vi "Read_write_p4.vi"() -> ()   [LabVIEW 2018]
uses:
  <instrlib>/LeCroy Wave Series/Public/Data/Read Single Waveform.vi
  <vilib>/Utility/file.llb/Read Delimited Spreadsheet (DBL).vi
  <vilib>/Utility/file.llb/Write Delimited Spreadsheet (DBL).vi
  <instrlib>/Siglent SDG X Series/Siglent SDG X Series.lvlib
  <instrlib>/LeCroy Wave Series/LeCroy Wave Series.lvlib
panel:
  in  "#Iteration":i32
  out "path":path
  out "error out 5":errorcluster
  out "error out 4":errorcluster
  out "resulting string":string
  out "#N_packet":i32
  out "error IO 2":errorcluster
  out "error IO":errorcluster
  in  "Read Directory":string
  out "error out 3":errorcluster
  in  "Write Directory":string
  in  "N_packets":i32
  in  "all rows 1":dbl[](array[numeric])
  in  "Tab Control":enum32{"Page 1", "Page 2"}(tab)
  in  "VISA Refnum in":refnum<visa-resource-name>
  in  "error in (no error)":errorcluster
  in  "Channel (1:Channel 1)":i32(ring)=1 items=["Channel 1"=1, "Channel 2"=2]
  in  "Enable Output (T: Enable)":bool=TRUE
  in  "Amplitude (1.0 Vpp)":dbl=1.0 format="%#.3f"
  in  "Frequency (1000 Hz)":dbl=1000.0 format="%#.6g"
  in  "DC Offset (0.00 V) in":dbl
  in  "Waveform Function (0: Sine) in":u16(ring) items=["Sine", "Square", "Ramp", "DC", "Pulse", "Arb"]
  in  "Phase (0.0 degrees)":dbl=0.002 min=-360.0 max=360.0 format="%#.1g"
  in  "Fall (20 ns)":dbl=2e-08 format="%#.3g"
  in  "Duty (20%)":dbl=4.32 min=0.0001 max=100.0 format="%.4g"
  in  "Delay (0.00 s)":dbl min=-1000000.0 max=1000000.0
  in  "Rise (20 ns)":dbl=1.04e-08 format="%#.3g"
  in  "True To \ngenerate\n pulse":bool
  out "VISA resource name out":refnum<visa-resource-name>
  out "error out":errorcluster
  in  "format string":string
  out "Output Filename":path
  out "error out 2":errorcluster
  in  "Filename":string="filename"
  in  "Path":string="c:\\path structure\\"
  in  "Read Directory":string
  out "Waveform Data":waveform(dbl)(graph)
  in  "Timeout (10000 ms)":u32=10000
  in  "Source (0: Channel 1)":u16(ring) items=["Channel 1", "Channel 2", "Channel 3", "Channel 4", "Memory 1", "Memory 2", "Memory 3", "Memory 4", "Function 1", "Function 2", "Function 3", "Function 4", "Function 5", "Function 6", "Function 7", "Function 8"]
  in  "Perform Auto Setup?":bool
  in  "Reset Scope?":bool
  in  "VISA resource name":refnum<visa-resource-name>
  out "Saved filename":string
  # "Set PULSE parameters"
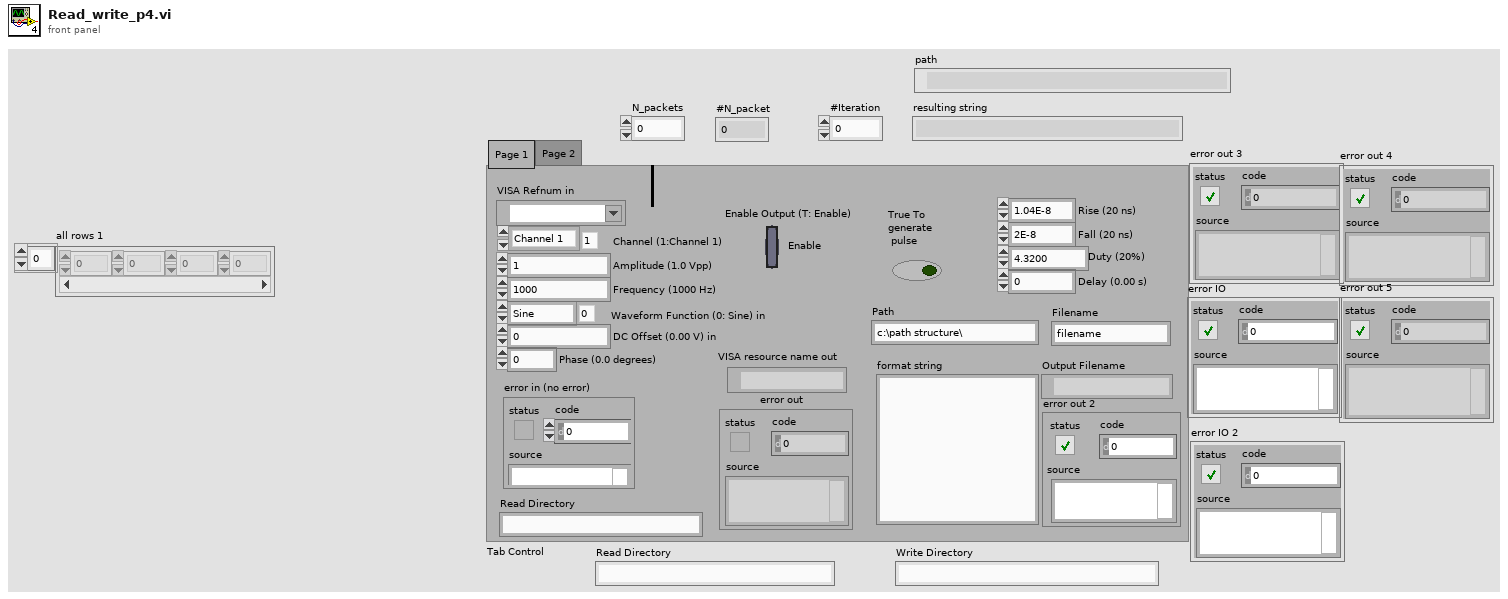
[diagram p1: front panel]
types:
  T1 = enum16{"open", "replace", "create", "open or create", "replace or create", "replace or create with confirmation"}
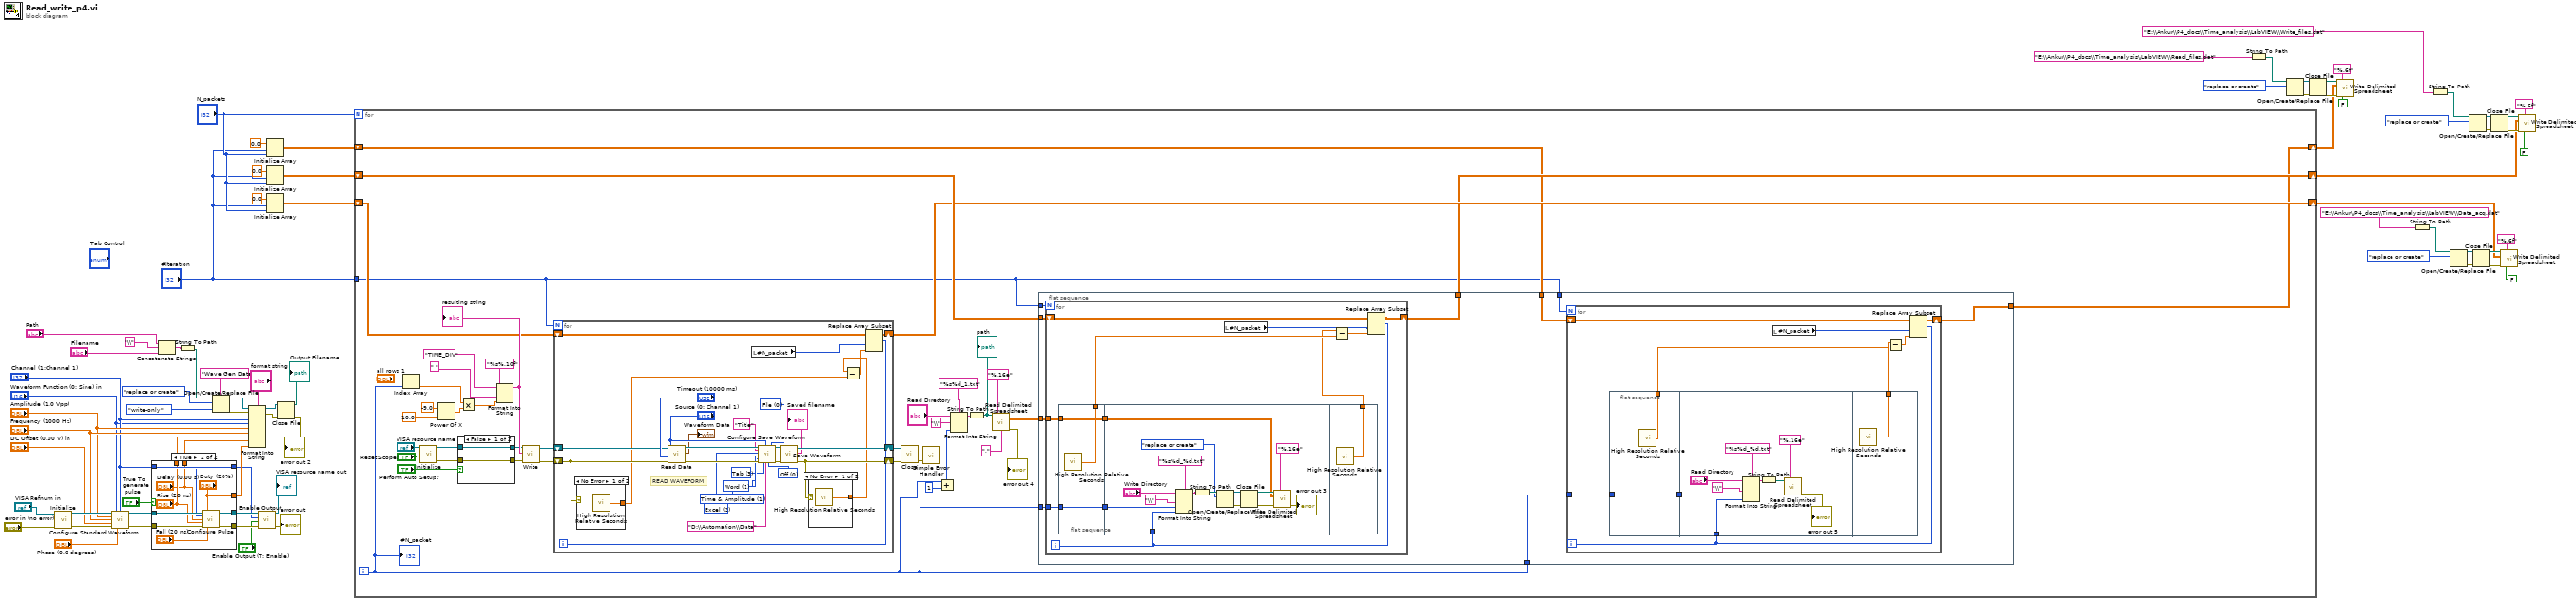
[diagram p0: block diagram]
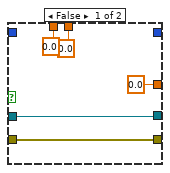
[diagram p2: hidden frame]
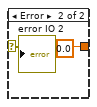
[diagram p3: hidden frame]
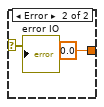
[diagram p4: hidden frame]
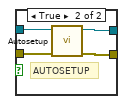
[diagram p5: hidden frame]
diagram:
  n1 = call <instrlib>:"Initialize.vi"("error in (no error)"="error in (no error)", "VISA resource name"="VISA Refnum in") -> ("error out"=w68:errorcluster, "VISA resource name out"=w69:refnum<visa-resource-name>)  [unwired: 8 in]
  n2 = call <instrlib>:"Configure Standard Waveform.vi"("VISA resource name"=w69, "Waveform Function (0: Sine)"="Waveform Function (0: Sine) in", "Channel (1:Channel 1)"="Channel (1:Channel 1)", "Amplitude (1.0 Vpp)"="Amplitude (1.0 Vpp)", "Frequency (1000 Hz)"="Frequency (1000 Hz)", "DC Offset (0.00 V)"="DC Offset (0.00 V) in", "error in (no error)"=w68, "Phase (0.0 degrees)"="Phase (0.0 degrees)") -> ("VISA resource name out"=w64:refnum<visa-resource-name>, "error out"=w67:errorcluster)  [unwired: 6 in]
  n3 = case shown="True" "True To \ngenerate\n pulse" {
    tunnel: [w79 w87] -> w74
    tunnel: [w78 w86] -> w73
    tunnel: w64 -> [w79 w85]
    tunnel: w67 -> [w78 w84]
    tunnel: "Channel (1:Channel 1)" -> [_ w83]
    tunnel: "Channel (1:Channel 1)" -> [_ _]
    tunnel: [0.0 ("Duty (20%)") "Duty (20%)"] -> w56
    tunnel: [0.0 ("Rise (20 ns)") "Rise (20 ns)"] -> w47
    tunnel: [0.0 ("Delay (0.00 s)") "Delay (0.00 s)"] -> w46
    frame False {
    }
    frame True {
      n4 = call <instrlib>:"Configure Pulse.vi"("VISA resource name"=w85, "Duty (20%)"="Duty (20%)", "Channel (1:Channel 1)"=w83, "Delay (0.00 s)"="Delay (0.00 s)", "Rise (20 ns)"="Rise (20 ns)", "error in (no error)"=w84, "Fall (20 ns)"="Fall (20 ns)") -> ("VISA resource name out"=w87:refnum<visa-resource-name>, "error out"=w86:errorcluster)  [unwired: 7 in]
    }
  }
  n5 = Concatenate Strings("Path", "\\" ("string"), "Filename") -> (w5:string)
  n6 = String To Path(string=w5) -> (path=w42:path)
  n7 = Open/Create/Replace File(file path (use dialog)=w42, prompt="Wave Gen Data", operation (0:open)=T1."replace or create", access (0:read/write)=enum16{"read/write", "read-only", "write-only"}."write-only") -> (refnum out=w58:refnum<file>, error out=w59:errorcluster)  [unwired: 2 in, 1 out]
  n8 = Format Into String(format string="format string", initial string=w58, error in=w59, "Channel (1:Channel 1)", "Waveform Function (0: Sine) in", "Amplitude (1.0 Vpp)", "Frequency (1000 Hz)", w47, w46, w56) -> (resulting string=w54:refnum<file>, error out=w51:errorcluster)
  n9 = call <instrlib>:"Enable Output.vi"("error in (no error)"=w73, "Enable Output (T: Enable)"="Enable Output (T: Enable)", "Channel (1:Channel 1)"="Channel (1:Channel 1)", "VISA resource name"=w74) -> ("error out"=→"error out":errorcluster, "VISA resource name out"=→"VISA resource name out":refnum<visa-resource-name>)  [unwired: 6 in]
  n10 = Initialize Array(0.0 ("element"), "#Iteration", "N_packets") -> (w36:dbl[][])
  n11 = Initialize Array(0.0 ("element"), "#Iteration", "N_packets") -> (w38:dbl[][])
  n12 = Initialize Array(0.0 ("element"), "#Iteration", "N_packets") -> (w37:dbl[][])
  n13 = Close File(refnum=w54, error in=w51) -> (path=→"Output Filename":path, error out=→"error out 2":errorcluster)
  n14 = for {
    N: "N_packets" -> [_]
    shift-right: [w93] -> w18
    shift-left: w38 -> [w100]
    shift-right: [w98] -> w9
    shift-left: w37 -> [w99]
    shift-right: [w91] -> w27
    shift-left: w36 -> [w92]
    tunnel: "#Iteration" -> [w90]
    i -> [w89]
    n15 = Index Array(array="all rows 1", index=w89) -> (element=w114:dbl)
    n16 = call <instrlib>:"Initialize.vi"("Reset? (T: Yes)"="Reset Scope?", "VISA resource name"="VISA resource name") -> ("error out"=w124:errorcluster, "VISA resource name out"=w123:refnum<visa-resource-name>)  [unwired: 8 in]
    n17 = Power Of X(1:10.0, 2:-9.0 ("y")) -> (0:w115:dbl)
    n18 = case shown="False" "Perform Auto Setup?" {
      tunnel: w124 -> [w223 w228]
      tunnel: w123 -> [w224 w227]
      tunnel: [w224 w226] -> w111
      tunnel: [w223 w225] -> w110
      frame False {
      }
      frame True {
        # "AUTOSETUP"
        n19 = call <instrlib>:"Autosetup.vi"("error in (no error)"=w228, "VISA resource name"=w227) -> ("error out"=w225:errorcluster, "VISA resource name out"=w226:refnum<visa-resource-name>)  [unwired: 8 in]
      }
    }
    n20 = Multiply(x=w114, y=w115) -> (x*y=w113:dbl)
    n21 = Format Into String(format string="%s%.10f", initial string="TIME_DIV", " " ("input 1"), w113) -> (resulting string=w112:string)  [unwired: 1 in, 1 out]
    "resulting string" <- w112
    n22 = call <instrlib>:"Write.vi"("error in (no error)"=w110, "Write Buffer"=w112, "VISA resource name"=w111) -> ("error out"=w108:errorcluster, "VISA resource name out"=w109:refnum<visa-resource-name>)  [unwired: 7 in]
    n23 = for {
      N: w90 -> [_]
      shift-right: [w216] -> w128
      shift-left: w109 -> [w200]
      shift-right: [w198] -> w129
      shift-left: w108 -> [w199]
      shift-right: [w191] -> w98
      shift-left: w99 -> [w194]
      i -> [w193]
      w204 = u16 3 items=["Comma", "Space", "Semicolon", "Tab"] ("Delimiter (  0:Comma)")
      w202 = u16 0 items=["Off", "Wrap", "Fill"] ("Auto Save (0:Off")
      w205 = u16 1 items=["Byte", "Word", "Auto"] ("BinarySubFormat (1: Word)")
      w206 = u16 1 items=["Amplitude Only", "Time & Amplitude", "With Header"] ("SubFormat (1: Time & Amplitude)")
      w207 = u16 2 items=["Binary", "ASCII", "Excel", "MATLAB", "MathCad", "WaveML"] ("Format (0: Binary)")
      w201 = u16 0 items=["File", "M1", "M2", "M3", "M4"] ("Destination (0:File)")
      # "READ WAVEFORM"
      n24 = case shown="No Error" w199 {
        selector: w199 -> [_ w222]
        tunnel: [w220 0.0] -> w195
        frame No Error {
          n25 = call <vilib>:"High Resolution Relative Seconds.vi"() -> ("relative seconds"=w220:dbl)
        }
        frame Error {
          "error IO" <- w222
        }
      }
      n26 = call-poly <instrlib>:"Read Data.vi"("error in (no error)"=w199, "Timeout (10000 ms)"="Timeout (10000 ms)", "Source (0: Channel 1)"="Source (0: Channel 1)", "VISA resource name"=w200) -> ("error out"=w211:errorcluster, "Waveform Data"=→"Waveform Data":waveform(dbl), "VISA resource name out"=w210:refnum<visa-resource-name>)  [unwired: 5 in]
      n27 = local read "#N_packet"() -> (w197:i32)
      n28 = call <instrlib>:"Configure Save Waveform.vi"("VISA resource name"=w210, "Trace Title (Title)"="Title", "Format (0: Binary)"=w207, "SubFormat (1: Time & Amplitude)"=w206, "BinarySubFormat (1: Word)"=w205, "error in (no error)"=w211, "Delimiter (  0:Comma)"=w204, "Source (0: Channel 1)"="Source (0: Channel 1)", "Save Files in Directory (D:\\Waveforms)"="D:\\Automation\\Data" ("Save Files in Directory (D:\\Waveforms)"), "Auto Save (0:Off"=w202, "Destination (0:File)"=w201) -> ("VISA resource name out"=w213:refnum<visa-resource-name>, "error out"=w214:errorcluster)  [unwired: 7 in]
      n29 = call <instrlib>:"Save Waveform.vi"("error in (no error)"=w214, "VISA resource name"=w213) -> ("error out"=w198:errorcluster, "Saved filename"=→"Saved filename":string, "VISA resource name out"=w216:refnum<visa-resource-name>)  [unwired: 7 in]
      n30 = case shown="No Error" w198 {
        selector: w198 -> [_ w219]
        tunnel: [w217 0.0] -> w196
        frame No Error {
          n31 = call <vilib>:"High Resolution Relative Seconds.vi"() -> ("relative seconds"=w217:dbl)
        }
        frame Error {
          "error IO 2" <- w219
        }
      }
      n32 = Subtract(x=w196, y=w195) -> (x-y=w192:dbl)
      n33 = Replace Array Subset(array=w194, new element=w192, index (row)=w193, index (col)=w197) -> (w191:dbl[][])
    }
    n34 = call <instrlib>:"Close.vi"("error in (no error)"=w129, "VISA resource name"=w128) -> ("error out"=w122:errorcluster)  [unwired: 9 in]
    n35 = call <vilib>:"Simple Error Handler.vi"("error in (no error)"=w122) -> ()  [unwired: 4 in, 5 out]
    n36 = Add(x=w89, y=1) -> (x+y=w94:i32)
    n37 = Format Into String(format string="%s%d_1.txt", initial string="Read Directory", "\\" ("input 1"), w94) -> (resulting string=w106:string)  [unwired: 1 in, 1 out]
    n38 = String To Path(string=w106) -> (path=w102:path)
    "path" <- w102
    n39 = call-poly <vilib>:"Read Delimited Spreadsheet.vi"("file path (dialog if empty)"=w102, "format (%.3f)"="%.16e", "delimiter (\\t)"="," ("delimiter (\\t)")) -> ("all rows"=w101:dbl[][], "error out"=→"error out 4":errorcluster)  [unwired: 7 in, 4 out]
    n40 = flat-sequence {
      tunnel: w101 -> [w134]
      tunnel: w100 -> [w133]
      tunnel: w89 -> [w132]
      tunnel: w90 -> [w131]
      tunnel: [w130] -> w93
      tunnel: w89 -> [w168]
      tunnel: w92 -> [w167]
      tunnel: [w166] -> w91
      tunnel: w90 -> [w165]
      frame #0 {
        n41 = for {
          N: w131 -> [_]
          tunnel: w132 -> [w145]
          shift-right: [w135] -> w130
          shift-left: w133 -> [w139]
          tunnel: w134 -> [w144]
          i -> [w137]
          n42 = flat-sequence {
            tunnel: w144 -> [w147]
            tunnel: w145 -> [w148]
            tunnel: [w148] -> w143
            tunnel: [w147] -> w142
            tunnel: [w146] -> w141
            tunnel: w137 -> [w151]
            tunnel: w143 -> [w158]
            tunnel: w142 -> [w150]
            tunnel: [w164] -> w140
            frame #0 {
              n43 = call <vilib>:"High Resolution Relative Seconds.vi"() -> ("relative seconds"=w146:dbl)
            }
            frame #1 {
              n44 = Format Into String(format string="%s%d_%d.txt", initial string="Write Directory", "\\" ("input 1"), w158, w151) -> (resulting string=w162:string)  [unwired: 1 in, 1 out]
              n45 = String To Path(string=w162) -> (path=w159:path)
              n46 = Open/Create/Replace File(file path (use dialog)=w159, operation (0:open)=T1."replace or create") -> (refnum out=w157:refnum<file>, error out=w156:errorcluster)  [unwired: 4 in, 1 out]
              n47 = Close File(refnum=w157, error in=w156) -> (path=w155:path, error out=w154:errorcluster)
              n48 = call-poly <vilib>:"Write Delimited Spreadsheet.vi"("file path (dialog if empty)"=w155, "format (%.3f)"="%.16e", "2D data"=w150, "error in (no error)"=w154) -> ("error out"=→"error out 3":errorcluster)  [unwired: 10 in, 1 out]
            }
            frame #2 {
              n49 = call <vilib>:"High Resolution Relative Seconds.vi"() -> ("relative seconds"=w164:dbl)
            }
          }
          n50 = local read "#N_packet"() -> (w138:i32)
          n51 = Subtract(x=w140, y=w141) -> (x-y=w136:dbl)
          n52 = Replace Array Subset(array=w139, new element=w136, index (row)=w137, index (col)=w138) -> (w135:dbl[][])
        }
      }
      frame #1 {
        n53 = for {
          N: w165 -> [_]
          tunnel: w168 -> [w177]
          shift-right: [w169] -> w166
          shift-left: w167 -> [w170]
          i -> [w171]
          n54 = flat-sequence {
            tunnel: w177 -> [w179]
            tunnel: [w179] -> w176
            tunnel: [w178] -> w173
            tunnel: w171 -> [w182]
            tunnel: w176 -> [w181]
            tunnel: [w189] -> w174
            frame #0 {
              n55 = call <vilib>:"High Resolution Relative Seconds.vi"() -> ("relative seconds"=w178:dbl)
            }
            frame #1 {
              n56 = Format Into String(format string="%s%d_%d.txt", initial string="Read Directory", "\\" ("input 1"), w181, w182) -> (resulting string=w187:string)  [unwired: 1 in, 1 out]
              n57 = String To Path(string=w187) -> (path=w183:path)
              n58 = call-poly <vilib>:"Read Delimited Spreadsheet.vi"("file path (dialog if empty)"=w183, "format (%.3f)"="%.16e") -> ("error out"=→"error out 5":errorcluster)  [unwired: 8 in, 5 out]
            }
            frame #2 {
              n59 = call <vilib>:"High Resolution Relative Seconds.vi"() -> ("relative seconds"=w189:dbl)
            }
          }
          n60 = local read "#N_packet"() -> (w172:i32)
          n61 = Subtract(x=w174, y=w173) -> (x-y=w175:dbl)
          n62 = Replace Array Subset(array=w170, new element=w175, index (row)=w171, index (col)=w172) -> (w169:dbl[][])
        }
      }
    }
    "#N_packet" <- w89
  }
  n63 = String To Path(string="E:\\Ankur\\P4_docs\\Time_analysis\\LabVIEW\\Read_files.dat" ("format string")) -> (path=w33:path)
  n64 = Open/Create/Replace File(file path (use dialog)=w33, operation (0:open)=T1."replace or create") -> (refnum out=w32:refnum<file>, error out=w31:errorcluster)  [unwired: 4 in, 1 out]
  n65 = Close File(refnum=w32, error in=w31) -> (path=w34:path, error out=w35:errorcluster)
  n66 = call-poly <vilib>:"Write Delimited Spreadsheet.vi"("file path (dialog if empty)"=w34, "format (%.3f)"="%.6f", "2D data"=w27, "error in (no error)"=w35, "transpose? (no:F)"=FALSE) -> ()  [unwired: 9 in, 2 out]
  n67 = String To Path(string="E:\\Ankur\\P4_docs\\Time_analysis\\LabVIEW\\Data_acq.dat" ("format string")) -> (path=w15:path)
  n68 = String To Path(string="E:\\Ankur\\P4_docs\\Time_analysis\\LabVIEW\\Write_files.dat" ("format string")) -> (path=w24:path)
  n69 = Open/Create/Replace File(file path (use dialog)=w15, operation (0:open)=T1."replace or create") -> (refnum out=w14:refnum<file>, error out=w13:errorcluster)  [unwired: 4 in, 1 out]
  n70 = Open/Create/Replace File(file path (use dialog)=w24, operation (0:open)=T1."replace or create") -> (refnum out=w23:refnum<file>, error out=w22:errorcluster)  [unwired: 4 in, 1 out]
  n71 = Close File(refnum=w14, error in=w13) -> (path=w16:path, error out=w17:errorcluster)
  n72 = Close File(refnum=w23, error in=w22) -> (path=w25:path, error out=w26:errorcluster)
  n73 = call-poly <vilib>:"Write Delimited Spreadsheet.vi"("file path (dialog if empty)"=w16, "format (%.3f)"="%.6f", "2D data"=w9, "error in (no error)"=w17, "transpose? (no:F)"=FALSE) -> ()  [unwired: 9 in, 2 out]
  n74 = call-poly <vilib>:"Write Delimited Spreadsheet.vi"("file path (dialog if empty)"=w25, "format (%.3f)"="%.6f", "2D data"=w18, "error in (no error)"=w26, "transpose? (no:F)"=FALSE) -> ()  [unwired: 9 in, 2 out]
